vi "401 Unauthorized.vi"() -> (3 "error":T1={"HTTP Code"=200, "JSON Response"={"error"="No Error", "reason"="No Error"}})   [LabVIEW 2016, in "ServerErrors.lvlib"]
uses:
  ServerErrors.lvlib
  Error Message--cluster.ctl
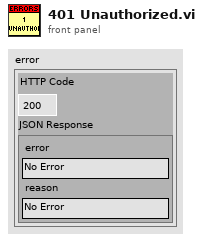
[diagram p1: front panel]
types:
  T1 = typedef "ServerErrors.lvlib/Error Message--cluster.ctl" = cluster{"HTTP Code":i32, "JSON Response":cluster{"error":string, "reason":string}}
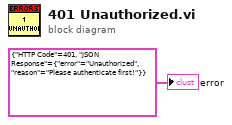
[diagram p0: block diagram]
diagram:
  "error" <- T1 {"HTTP Code"=401, "JSON Response"={"error"="Unauthorized", "reason"="Please authenticate first!"}} ("error")
